vi "LVClass_Camera write camera.vi"(8 "error in (no error)":errorcluster, 10 "camera":i32, 11 "Camera in":refnum<class "Camera.lvclass">) -> (0 "error out":errorcluster, 3 "Camera out":refnum<class "Camera.lvclass">)   [LabVIEW 2020, in "Camera.lvclass"]
uses:
  Camera.lvclass
  Handle creation.ctl
  Camera.lvclass/Camera.ctl
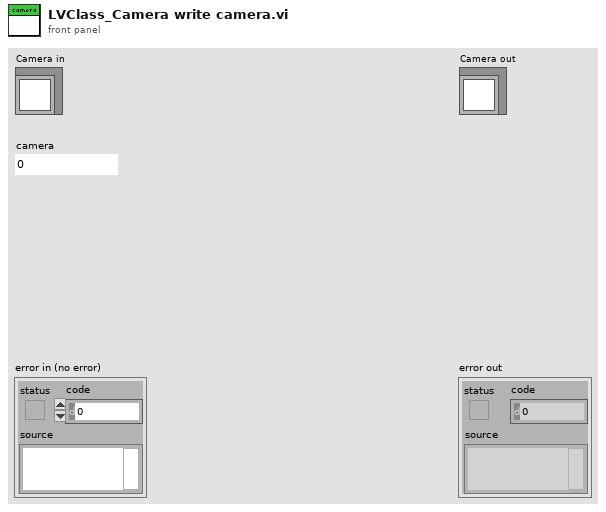
[diagram p1: front panel]
types:
  T1 = typedef "Handle creation.ctl" = enum16{"By ctor", "By write function"}
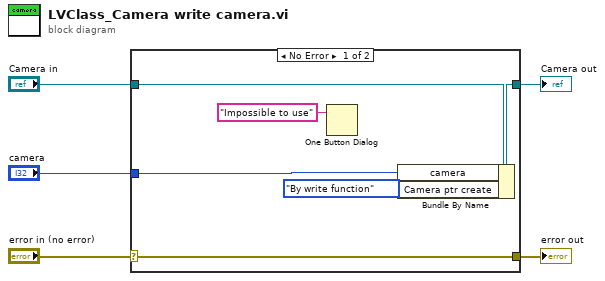
[diagram p0: block diagram]
diagram:
  n1 = case shown="No Error" "error in (no error)" {
    selector: "error in (no error)" -> [w11 w12]
    tunnel: [w11 w12] -> w4
    tunnel: [w9 w13] -> w2
    tunnel: "Camera in" -> [w10 w13]
    tunnel: "camera" -> [w8 _]
    frame No Error {
      n2 = One Button Dialog(message="Impossible to use") -> ()  [unwired: 1 in, 1 out]
      n3 = Bundle By Name(cluster=w10, "camera"=w8, "Camera ptr create"=Handle_creation."By write function") -> (w9:refnum<class "Camera.lvclass">)
    }
    frame Error {
    }
  }
  "error out" <- w4
  "Camera out" <- w2
